vi "base64url Encode.vi"(7 "Padding (F)":bool, 11 "String":string) -> (3 "base64url":string)   [LabVIEW 2019, in "Base64 Support.lvlib"]
uses:
  Base64 Support.lvlib
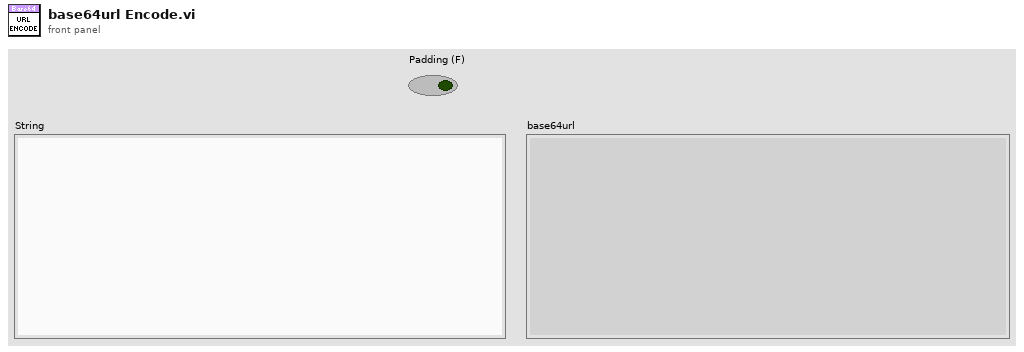
[diagram p1: front panel]
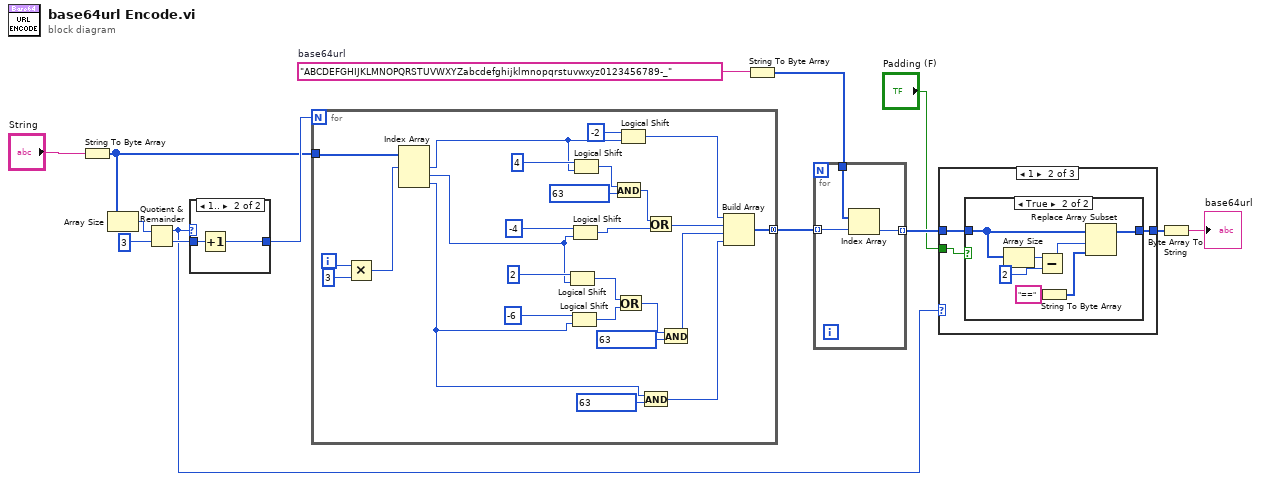
[diagram p0: block diagram]
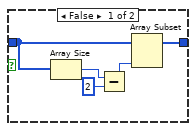
[diagram p3: hidden frame]
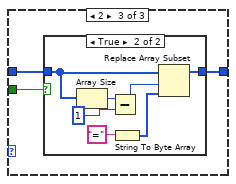
[diagram p4: hidden frame]
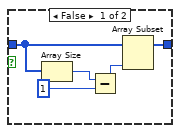
[diagram p5: hidden frame]
diagram:
  w14 = "ABCDEFGHIJKLMNOPQRSTUVWXYZabcdefghijklmnopqrstuvwxyz0123456789-_"  # base64url
  n1 = String To Byte Array(string="String") -> (unsigned byte array=w9:u8[])
  n2 = Array Size(array=w9) -> (size(s)=w11:i32)
  n3 = Quotient & Remainder(x=w11, y=3) -> (x-y*floor(x/y)=w2:i32, floor(x/y)=w5:i32)
  n4 = case shown="1.." w2 {
    tunnel: w5 -> [w15 w17]
    tunnel: [w15 w16] -> w10
    frame ..0 {
    }
    frame 1.. {
      n5 = Increment(x=w17) -> (x+1=w16:i32)
    }
  }
  n6 = for {
    N: w10 -> [_]
    tunnel: w9 -> [w41]
    tunnel: [w33] -> w8 mode=concatenating
    i -> [w43]
    n7 = Multiply(x=w43, y=3) -> (x*y=w39:i32)
    n8 = Index Array(array=w41, index #1=w39) -> (element #1=w35:u8, element #2=w31:u8, element #3=w20:u8)  [unwired: 2 in]
    n9 = Logical Shift(y=i16 2, x=w31) -> (x << y=w25:u8)
    n10 = Logical Shift(y=i16 -6, x=w20) -> (x << y=w24:u8)
    n11 = Logical Shift(y=i16 -4, x=w31) -> (x << y=w36:u8)
    n12 = Logical Shift(y=i16 4, x=w35) -> (x << y=w28:u8)
    n13 = And(x=w28, y=u8 63) -> (x .and. y?=w27:u8)
    n14 = Or(x=w25, y=w24) -> (x .or. y?=w22:u8)
    n15 = Logical Shift(y=i16 -2, x=w35) -> (x << y=w34:u8)
    n16 = And(x=w20, y=u8 63) -> (x .and. y?=w18:u8)
    n17 = Or(x=w27, y=w36) -> (x .or. y?=w30:u8)
    n18 = And(x=w22, y=u8 63) -> (x .and. y?=w21:u8)
    n19 = Build Array(w34, w30, w21, w18) -> (w33:u8[])
  }
  n20 = String To Byte Array(string=w14) -> (unsigned byte array=w7:u8[])
  n21 = for {
    tunnel: w8 -> [w46] mode=indexing
    tunnel: w7 -> [w45]
    tunnel: [w44] -> w4 mode=indexing
    n22 = Index Array(array=w45, index=w46) -> (element=w44:u8)
  }
  n23 = case shown="1" w2 {
    tunnel: w4 -> [w47 w50 w65]
    tunnel: [w47 w49 w64] -> w3
    tunnel: "Padding (F)" -> [_ w48 w63]
    frame 0, Default {
    }
    frame 1 {
      n24 = case shown="True" w48 {
        tunnel: w50 -> [w55 w57]
        tunnel: [w52 w56] -> w49
        frame False {
          n25 = Array Size(array=w55) -> (size(s)=w54:i32)
          n26 = Subtract(x=w54, y=2) -> (x-y=w51:i32)
          n27 = Array Subset(array=w55, length=w51) -> (w52:u8[])  [unwired: 1 in]
        }
        frame True {
          n28 = Array Size(array=w57) -> (size(s)=w62:i32)
          n29 = Subtract(x=w62, y=2) -> (x-y=w60:i32)
          n30 = String To Byte Array(string="==") -> (unsigned byte array=w58:u8[])
          n31 = Replace Array Subset(array=w57, new element=w58, index=w60) -> (w56:u8[])
        }
      }
    }
    frame 2 {
      n32 = case shown="True" w63 {
        tunnel: w65 -> [w70 w77]
        tunnel: [w67 w74] -> w64
        frame False {
          n33 = Array Size(array=w70) -> (size(s)=w69:i32)
          n34 = Subtract(x=w69, y=1) -> (x-y=w66:i32)
          n35 = Array Subset(array=w70, length=w66) -> (w67:u8[])  [unwired: 1 in]
        }
        frame True {
          n36 = Array Size(array=w77) -> (size(s)=w76:i32)
          n37 = Subtract(x=w76, y=1) -> (x-y=w73:i32)
          n38 = String To Byte Array(string="=") -> (unsigned byte array=w71:u8[])
          n39 = Replace Array Subset(array=w77, new element=w71, index=w73) -> (w74:u8[])
        }
      }
    }
  }
  n40 = Byte Array To String(unsigned byte array=w3) -> (string=→"base64url":string)
